vi "Pre Launch Init.vi"(11 "HTTP发送 in":refnum<class "HTTP发送.lvclass"> caption="操作者输入") -> (0 "error out":errorcluster caption="错误输出", 3 "HTTP发送 out":refnum<class "HTTP发送.lvclass"> caption="操作者输出")   [LabVIEW 2016, in "工况数据上传.lvlib" / "HTTP发送.lvclass"]
doc: "(<B>Filename</B>: Actor Framework.lvlib:Actor.lvclass:Pre Launch Init.vi)\n\nDefines behavior that occurs after the Launch Nested Actor method is invoked but before the actor's Actor Core method begins running.\n\nBy default, this method does nothing.子孙类重写该方法定义具体的操作。"
uses:
  <vilib>/ActorFramework/Actor/Actor.lvclass
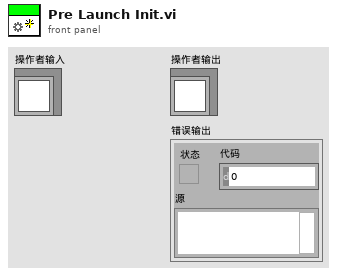
[diagram p1: front panel]
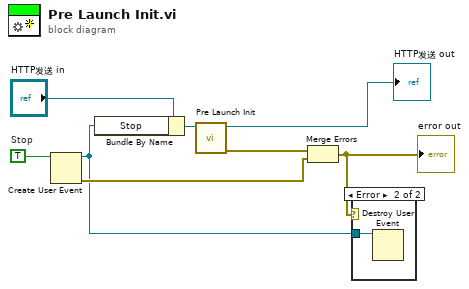
[diagram p0: block diagram]
diagram:
  w7 = TRUE  # Stop
  n1 = Create User Event(user event datatype=w7) -> (user event=w2:refnum<user-event>, error out=w3:errorcluster)  [unwired: 1 in]
  n2 = Bundle By Name(cluster="HTTP发送 in", "Stop"=w2) -> (w5:refnum<class "HTTP发送.lvclass">)
  n3 = call-parent "Pre Launch Init.vi"("Actor in"=w5) -> ("error out"=w4:errorcluster, "Actor out"=→"HTTP发送 out":refnum<class "HTTP发送.lvclass">)  [unwired: 9 in]
  n4 = Merge Errors(w4, w3) -> (w1:errorcluster)
  "error out" <- w1
  n5 = case shown="Error" w1 {
    tunnel: w2 -> [_ w9]
    frame No Error {
    }
    frame Error {
      n6 = Destroy User Event(user event=w9) -> ()  [unwired: 1 in, 1 out]
    }
  }
